vi "write data.vi"() -> ()   [LabVIEW 2025]
uses:
  Classes/data log/data log.lvclass
  <vilib>/numeric/Random Number (Range) DBL.vi
panel:
  out "error out 2":errorcluster
  out "error out":errorcluster
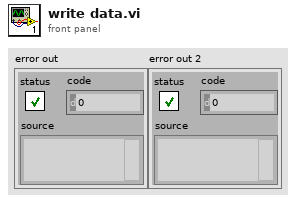
[diagram p1: front panel]
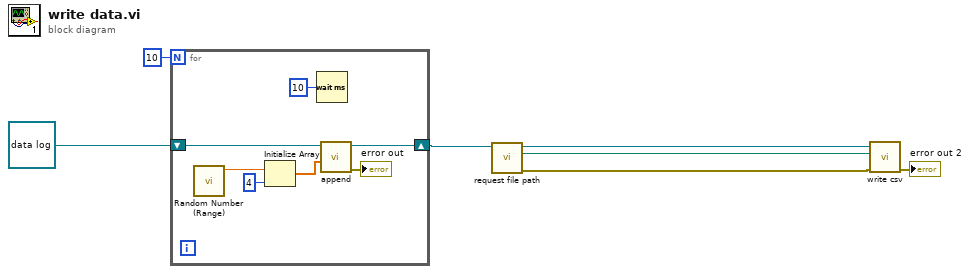
[diagram p0: block diagram]
diagram:
  n1 = for {
    N: 10 -> [_]
    shift-right: [w13] -> w4
    shift-left: refnum<class "data log.lvclass"> refnum ("data log.lvclass") -> [w14]
    n2 = call-poly <vilib>:"Random Number (Range).vi"() -> ("number"=w12:dbl)  [unwired: 11 in]
    n3 = Initialize Array(w12, 4 ("dimension size")) -> (w10:dbl[])
    n4 = Wait (ms)(milliseconds to wait=u32 10) -> ()  [unwired: 1 out]
    n5 = call-dynamic "append.vi"("data"=w10, "data log in"=w14) -> ("error out"=→"error out":errorcluster, "data log out"=w13:refnum<class "data log.lvclass">)  [unwired: 8 in]
  }
  n6 = call-dynamic "request file path.vi"("data log in"=w4) -> ("error out"=w1:errorcluster, "selected path"=w2:path, "data log out"=w3:refnum<class "data log.lvclass">)  [unwired: 8 in]
  n7 = call-dynamic "write csv.vi"("error in (no error)"=w1, "file path (dialog if empty)"=w2, "data log in"=w3) -> ("error out"=→"error out 2":errorcluster)  [unwired: 7 in, 1 out]
